vi "test_VariousDataTypes_GetParameterInformation_MatchesExpectedInformation.vi"(8 "error in":errorcluster) -> (0 "error out":errorcluster, 2 "result":string, 3 "pass":bool)   [LabVIEW 2020, in "MeasurementServerTests.lvlib"]
uses:
  MeasurementServerTests.lvlib
  Runtime/MeasurementLink Measurement Server/Helpers/TypeDefs/google_protobuf_Field_Kind.ctl
  gRPC/Generated APIs/ni/protobuf/types/RPC Messages/ni_protobuf_types_DoubleXYData.ctl
  Runtime/MeasurementLink Measurement Server/MeasurementLink Measurement Server.lvlib
  <vilib>/Utility/Data Type/NI_Data Type.lvlib
  gRPC/Generated APIs/ni/protobuf/types/ni.protobuf.types.lvlib
panel:
  out "actual results":T2(array[cluster])=[{"name"="double", "Kind"=enum."TYPE_DOUBLE", "repeated"=FALSE, "message_type"=""}, {"name"="int64", "Kind"=enum."TYPE_INT64", "repeated"=FALSE, "message_type"=""}, {"name"="uint64", "Kind"=enum."TYPE_UINT64", "repeated"=FALSE, "message_type"=""}, {"name"="int32", "Kind"=enum."TYPE_INT32", "repeated"=FALSE, "message_type"=""}, {"name"="uint32", "Kind"=enum."TYPE_UINT32", "repeated"=FALSE, "message_type"=""}, {"name"="int16", "Kind"=enum."TYPE_UNKNOWN", "repeated"=FALSE, "message_type"=""}, {"name"="uint16", "Kind"=enum."TYPE_UNKNOWN", "repeated"=FALSE, "message_type"=""}, {"name"="bool", "Kind"=enum."TYPE_BOOL", "repeated"=FALSE, "message_type"=""}, {"name"="string", "Kind"=enum."TYPE_STRING", "repeated"=FALSE, "message_type"=""}, {"name"="double array", "Kind"=enum."TYPE_DOUBLE", "repeated"=TRUE, "message_type"=""}, {"name"="uint64 array", "Kind"=enum."TYPE_UINT64", "repeated"=TRUE, "message_type"=""}, {"name"="ni_protobuf_types_DoubleXYData", "Kind"=enum."TYPE_MESSAGE", "repeated"=FALSE, "message_type"="ni.protobuf.types.DoubleXYData"}, {"name"="cluster of double", "Kind"=enum."TYPE_UNKNOWN", "repeated"=FALSE, "message_type"=""}]
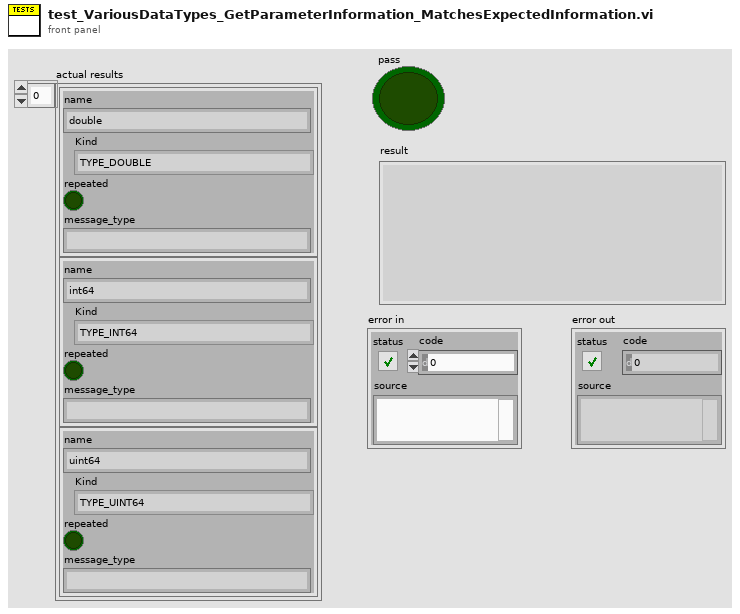
[diagram p1: front panel]
types:
  T1 = typedef "MeasurementLink Measurement Server.lvlib/google_protobuf_Field_Kind.ctl" = enum32{"TYPE_UNKNOWN", "TYPE_DOUBLE", "TYPE_FLOAT", "TYPE_INT64", "TYPE_UINT64", "TYPE_INT32", "TYPE_FIXED64", "TYPE_FIXED32", "TYPE_BOOL", "TYPE_STRING", "TYPE_GROUP", "TYPE_MESSAGE", "TYPE_BYTES", "TYPE_UINT32", "TYPE_ENUM", "TYPE_SFIXED32", "TYPE_SFIXED64", "TYPE_SINT32", "TYPE_SINT64"}
  T2 = cluster{"name":string, "Kind":T1, "repeated":bool, "message_type":string}[]
  T3 = typedef "ni.protobuf.types.lvlib/ni_protobuf_types_DoubleXYData.ctl" = cluster{"x_data":dbl[], "y_data":dbl[]}
  T4 = cluster{"double":dbl, "int64":i64, "uint64":u64, "int32":i32, "uint32":u32, "int16":i16, "uint16":u16, "bool":bool, "string":string, "double array":dbl[], "uint64 array":u64[], "ni_protobuf_types_DoubleXYData":T3, "cluster of double":cluster{"Numeric":dbl}, "enum u32":enum32{""}, "enum u16":enum16{""}, "enum u8":enum8{""}}
  T5 = cluster{"name":string, "Kind":T1, "repeated":bool, "message_type":string}
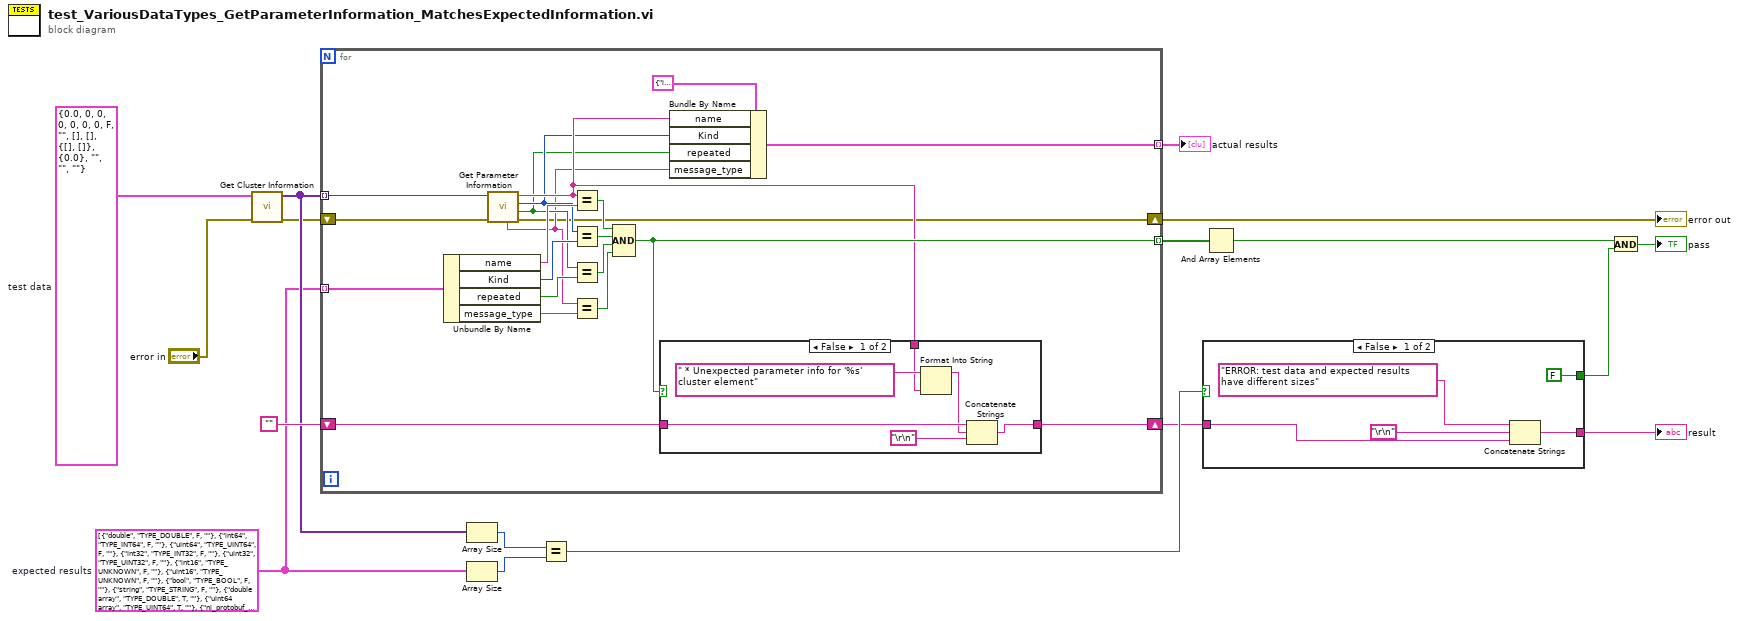
[diagram p0: block diagram]
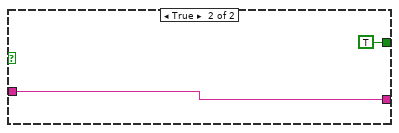
[diagram p2: hidden frame]
diagram:
  w4 = T2 [{"name"="double", "Kind"=enum."TYPE_DOUBLE", "repeated"=FALSE, "message_type"=""}, {"name"="int64", "Kind"=enum."TYPE_INT64", "repeated"=FALSE, "message_type"=""}, {"name"="uint64", "Kind"=enum."TYPE_UINT64", "repeated"=FALSE, "message_type"=""}, {"name"="int32", "Kind"=enum."TYPE_INT32", "repeated"=FALSE, "message_type"=""}, {"name"="uint32", "Kind"=enum."TYPE_UINT32", "repeated"=FALSE, "message_type"=""}, {"name"="int16", "Kind"=enum."TYPE_UNKNOWN", "repeated"=FALSE, "message_type"=""}, {"name"="uint16", "Kind"=enum."TYPE_UNKNOWN", "repeated"=FALSE, "message_type"=""}, {"name"="bool", "Kind"=enum."TYPE_BOOL", "repeated"=FALSE, "message_type"=""}, {"name"="string", "Kind"=enum."TYPE_STRING", "repeated"=FALSE, "message_type"=""}, {"name"="double array", "Kind"=enum."TYPE_DOUBLE", "repeated"=TRUE, "message_type"=""}, {"name"="uint64 array", "Kind"=enum."TYPE_UINT64", "repeated"=TRUE, "message_type"=""}, {"name"="ni_protobuf_types_DoubleXYData", "Kind"=enum."TYPE_MESSAGE", "repeated"=FALSE, "message_type"="ni.protobuf.types.DoubleXYData"}, {"name"="cluster of double", "Kind"=enum."TYPE_UNKNOWN", "repeated"=FALSE, "message_type"=""}, {"name"="enum u32", "Kind"=enum."TYPE_ENUM", "repeated"=FALSE, "message_type"=""}, {"name"="enum u16", "Kind"=enum."TYPE_UNKNOWN", "repeated"=FALSE, "message_type"=""}, {"name"="enum u8", "Kind"=enum."TYPE_UNKNOWN", "repeated"=FALSE, "message_type"=""}]  # expected results
  w5 = T4 {"double"=0.0, "int64"=0, "uint64"=0, "int32"=0, "uint32"=0, "int16"=0, "uint16"=0, "bool"=FALSE, "string"="", "double array"=[], "uint64 array"=[], "ni_protobuf_types_DoubleXYData"={"x_data"=[], "y_data"=[]}, "cluster of double"={"Numeric"=0.0}, "enum u32"=enum."", "enum u16"=enum."", "enum u8"=enum.""}  # test data
  n1 = call <vilib>:"Get Cluster Information.vi"("error in (no error)"="error in", "variant"=w5) -> ("error out"=w2:errorcluster, "cluster elements"=w15:variant[])  [unwired: 8 in]
  n2 = for {
    tunnel: w4 -> [w37] mode=indexing
    tunnel: w15 -> [w38] mode=indexing
    tunnel: [w28] -> w17 mode=indexing
    shift-right: [w26] -> w10
    shift-left: "" -> [w27]
    tunnel: [w20] -> w6 mode=indexing
    shift-right: [w18] -> w1
    shift-left: w2 -> [w19]
    n3 = Unbundle By Name(w37) -> ("name"=w36:string, "Kind"=w35:T1, "repeated"=w34:bool, "message_type"=w33:string)
    n4 = call "Get Parameter Information.vi"("error in (no error)"=w19, "variant data"=w38) -> ("error out"=w18:errorcluster, "repeated"=w22:bool, "grpc_type"=w23:T1, "name"=w24:string, "message_type"=w21:string)  [unwired: 5 in]
    n5 = Equal?(x=w24, y=w36) -> (x = y?=w32:bool)
    n6 = Equal?(x=w23, y=w35) -> (x = y?=w31:bool)
    n7 = Equal?(x=w22, y=w34) -> (x = y?=w30:bool)
    n8 = Equal?(x=w21, y=w33) -> (x = y?=w29:bool)
    n9 = Compound Arithmetic op=AND(w32, w31, w30, w29) -> (w28:bool)
    n10 = case shown="False" w28 {
      tunnel: w24 -> [w43 _]
      tunnel: w27 -> [w42 w45]
      tunnel: [w39 w45] -> w26
      frame False {
        n11 = Format Into String(format string=" * Unexpected parameter info for '%s' cluster element", w43) -> (resulting string=w41:string)  [unwired: 2 in, 1 out]
        n12 = Concatenate Strings(w42, w41, "\r\n") -> (w39:string)
      }
      frame True {
      }
    }
    n13 = Bundle By Name(cluster=T5 {"name"="int32", "Kind"=enum."TYPE_SINT32", "repeated"=FALSE, "message_type"=""} ("Cluster"), "name"=w24, "Kind"=w23, "repeated"=w22, "message_type"=w21) -> (w20:T5)
  }
  "error out" <- w1
  "actual results" <- w6
  n14 = Array Size(array=w15) -> (size(s)=w14:i32)
  n15 = Array Size(array=w4) -> (size(s)=w13:i32)
  n16 = Equal?(x=w14, y=w13) -> (x = y?=w12:bool)
  n17 = case shown="False" w12 {
    tunnel: w10 -> [w46 w52]
    tunnel: [w50 w52] -> w11
    tunnel: [FALSE TRUE] -> w8
    frame False {
      n18 = Concatenate Strings("ERROR: test data and expected results have different sizes", "\r\n", w46) -> (w50:string)
    }
    frame True {
    }
  }
  "result" <- w11
  n19 = And Array Elements(Boolean array=w17) -> (logical AND=w9:bool)
  n20 = And(x=w9, y=w8) -> (x .and. y?=→"pass":bool)
